vi "Read Callibration Datas.vi"(8 "error in (no error)":errorcluster, 11 "file (use dialog)":path=path "D:/WeiFu/Labview ATS/Corner Radar/EOL Test/Corner EOL Radar ATS/SubVi/C Lib/20250509/data_.txt") -> (0 "error out":errorcluster, 3 "Datas":T1[](array[typedef]))   [LabVIEW 2024]
uses:
  Controls/calculate_doa_struct.ctl
  Controls/ant re&im.ctl
  Controls/Calc Para_int.ctl
  Controls/Calc Para_float.ctl
panel:
  out "Numeric":i32
  out "array type (2D Dbl) 2":dbl[](array[numeric])
  out "array type (2D Dbl)":dbl[][](array[numeric])
  out "size(s)":i32
  out "x/y":dbl
  out "array":dbl[](array[numeric])
  out "text":string
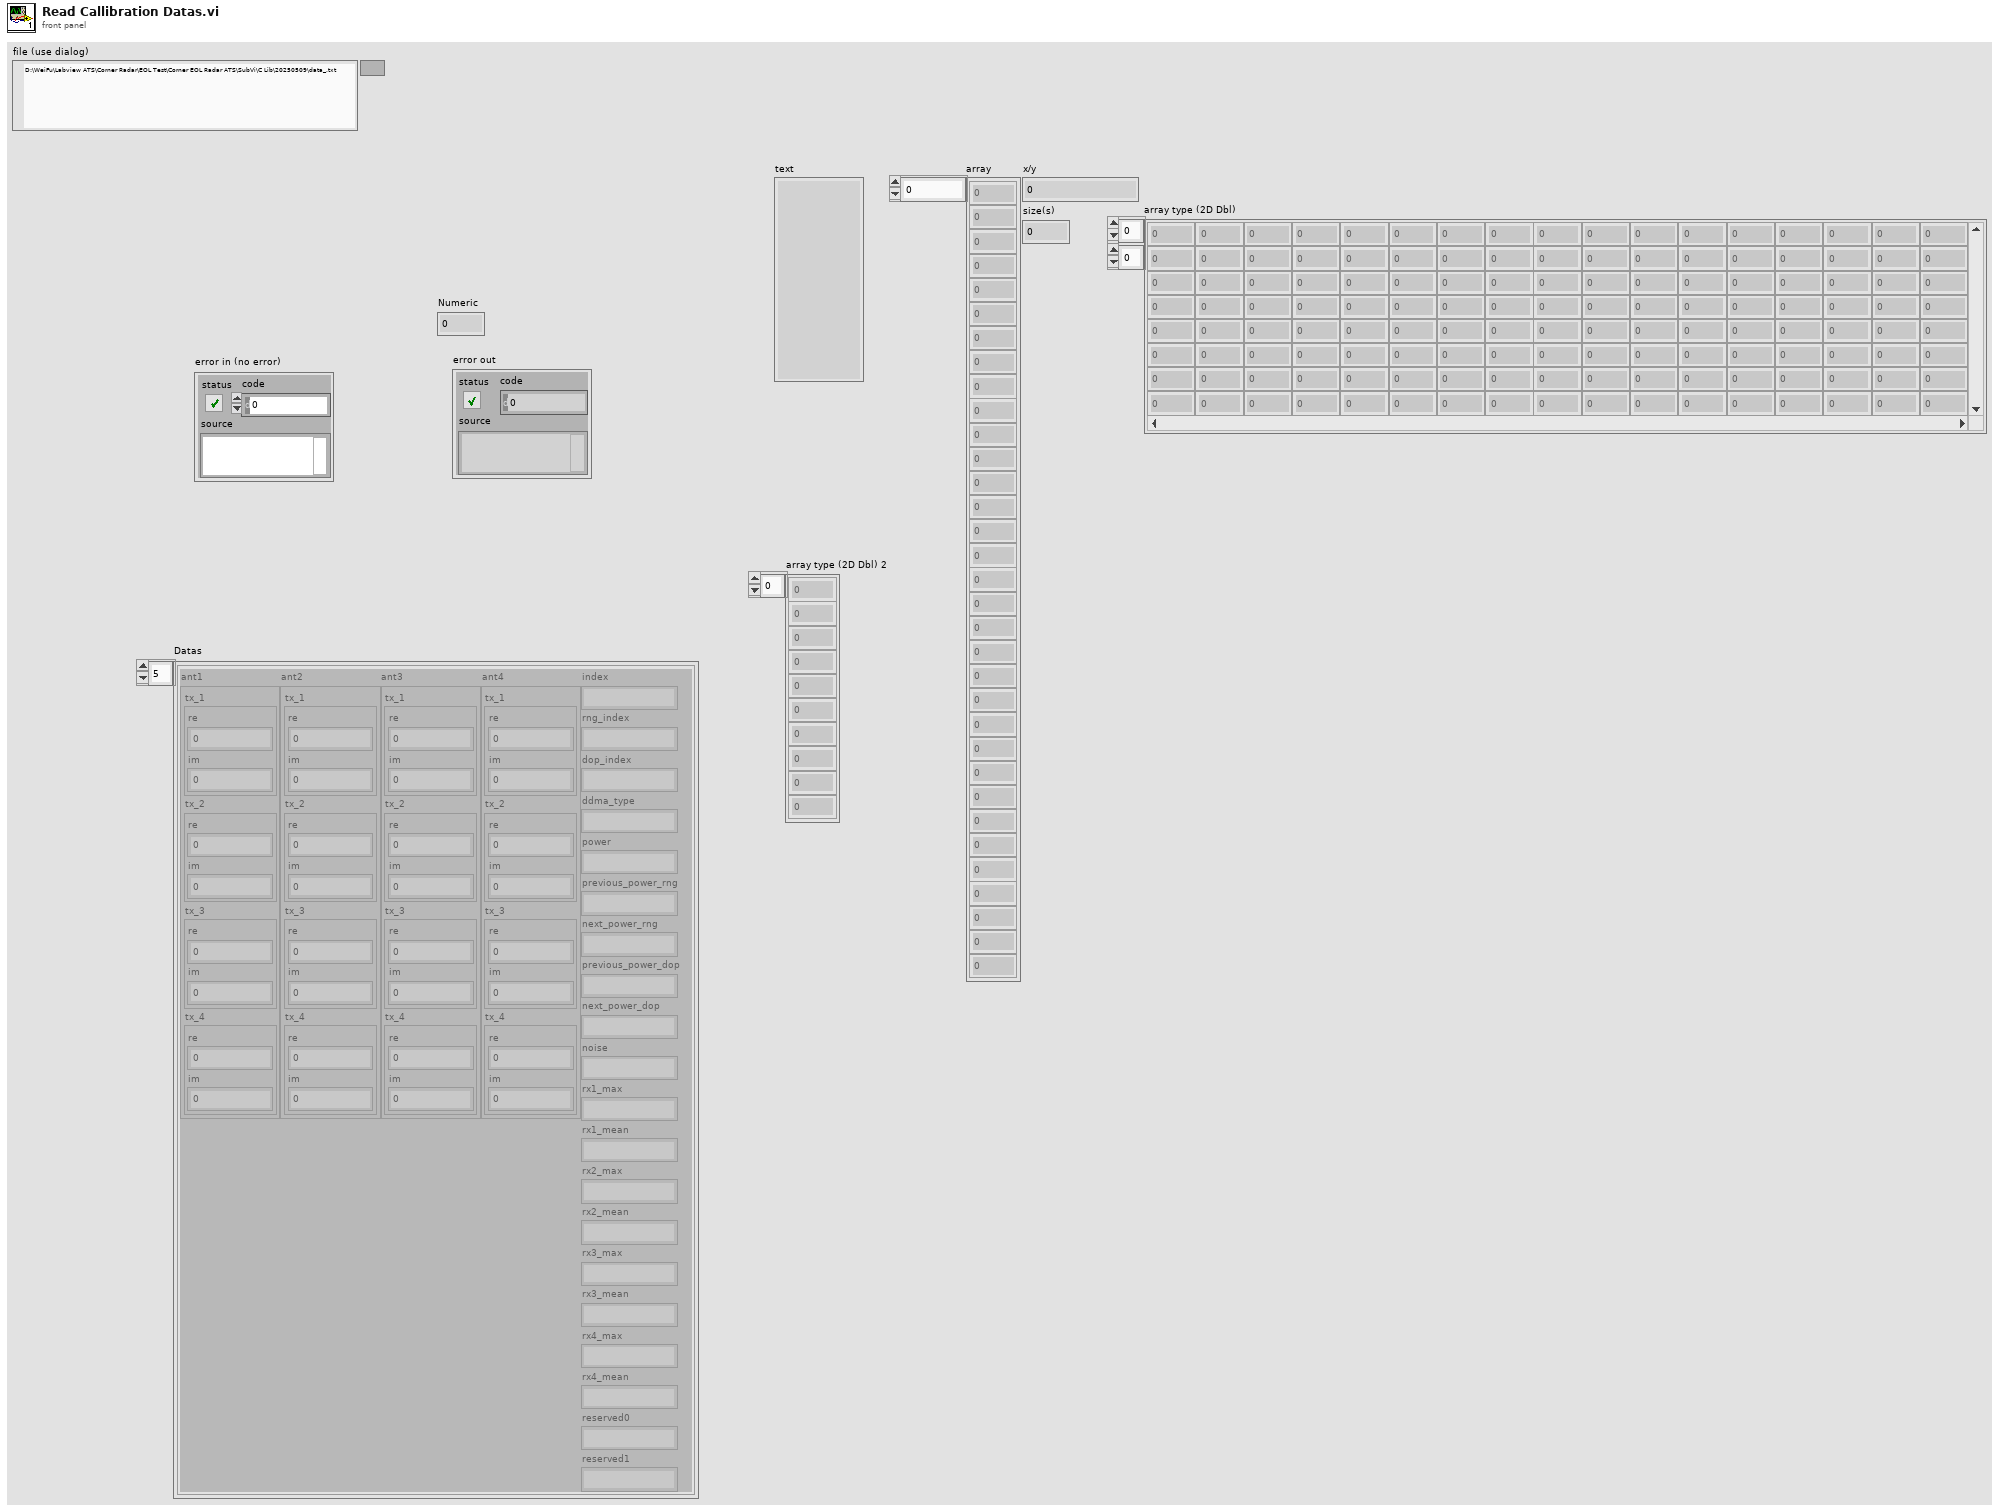
[diagram p1: front panel]
types:
  T1 = typedef "calculate_doa_struct.ctl" = cluster{"ant1":T2, "ant2":T2, "ant3":T2, "ant4":T2, "index":u16, "rng_index":u16, "dop_index":u16, "ddma_type":u16, "power":u32, "previous_power_rng":u32, "next_power_rng":u32, "previous_power_dop":u32, "next_power_dop":u32, "noise":u32, "rx1_max":u32, "rx1_mean":u32, "rx2_max":u32, "rx2_mean":u32, "rx3_max":u32, "rx3_mean":u32, "rx4_max":u32, "rx4_mean":u32, "reserved0":u32, "reserved1":u32}
  T2 = typedef "ant re&im.ctl" = cluster{"tx_1":T3, "tx_2":T3, "tx_3":T3, "tx_4":T3}
  T3 = typedef "Calc Para_int.ctl" = cluster{"re":i32, "im":i32}
  T4 = cluster{"tx_0":T3, "tx_1":T3, "tx_2":T3, "tx_3":T3}
  T5 = typedef "Calc Para_float.ctl" = cluster{"re":sgl, "im":sgl}
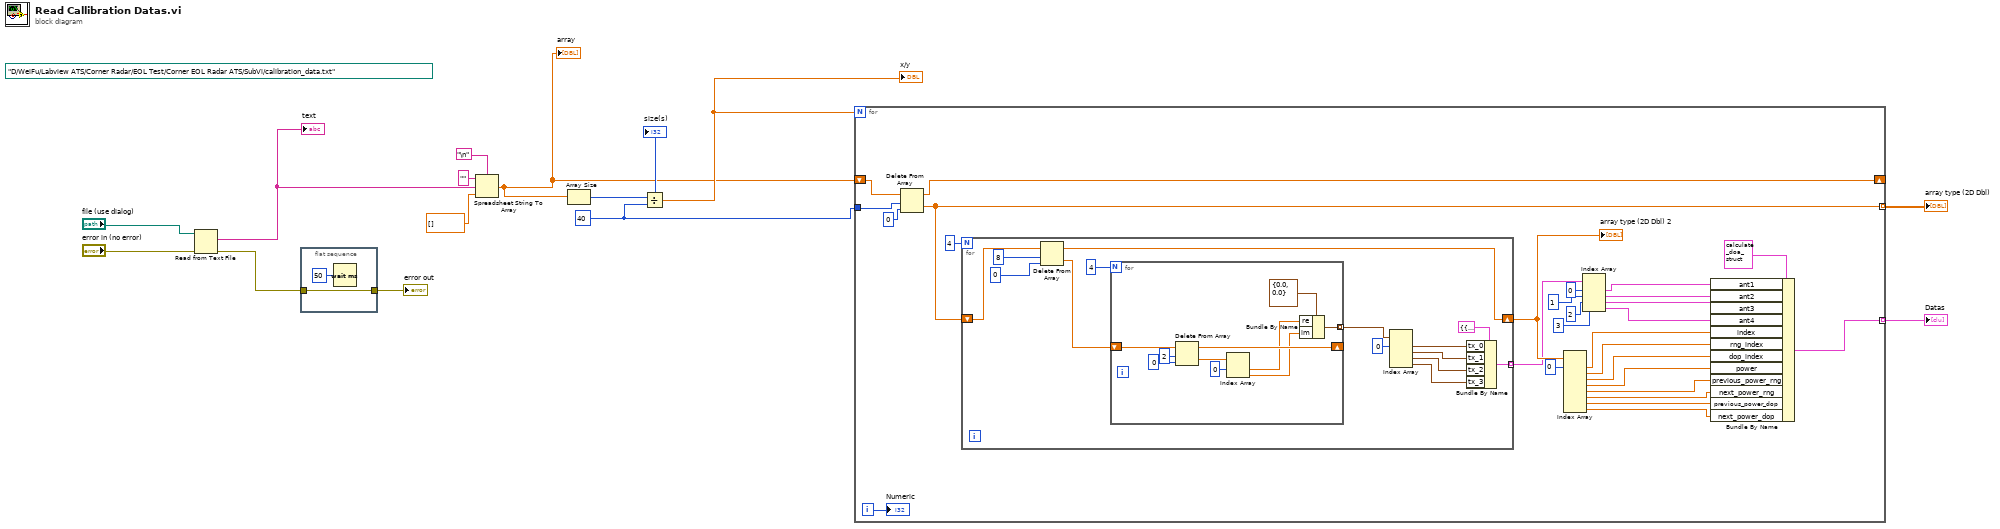
[diagram p0: block diagram]
diagram:
  w7 = 40 ("y")
  (unwired) path "D:/WeiFu/Labview ATS/Corner Radar/EOL Test/Corner EOL Radar ATS/SubVi/calibration_data.txt" ("file (use dialog)")
  n1 = Read from Text File(file (use dialog)="file (use dialog)", error in="error in (no error)") -> (text=w14:string, error out=w3:errorcluster)  [unwired: 2 in, 2 out]
  "text" <- w14
  n2 = flat-sequence {
    tunnel: w3 -> [w15]
    tunnel: [w15] -> w1
    frame #0 {
      n3 = Wait (ms)(milliseconds to wait=u32 50) -> ()  [unwired: 1 out]
    }
  }
  n4 = Spreadsheet String To Array(delimiter (Tab)="\n", format string="", spreadsheet string=w14, array type (2D Dbl)=dbl[] []) -> (array=w8:dbl[])
  "array" <- w8
  n5 = Array Size(array=w8) -> (size(s)=w10:i32)
  "size(s)" <- w10
  n6 = Divide(x=w10, y=w7) -> (x/y=w9:dbl)
  "x/y" <- w9
  n7 = for {
    N: w9 -> [_]
    shift-right: [w41] -> _
    shift-left: w8 -> [w44]
    tunnel: w7 -> [w43]
    tunnel: [w39] -> w6 mode=indexing
    tunnel: [w40] -> w5 mode=indexing
    i -> [w17]
    n8 = Delete From Array(array=w44, length=w43, index=0) -> (deleted portion=w39:dbl[], array with subset deleted=w41:dbl[])
    n9 = for {
      N: 4 -> [_]
      shift-right: [w55] -> w38
      shift-left: w39 -> [w56]
      tunnel: [w46] -> w35 mode=indexing
      n10 = Delete From Array(array=w56, length=8, index=0) -> (deleted portion=w53:dbl[], array with subset deleted=w55:dbl[])
      n11 = for {
        N: 4 -> [_]
        shift-right: [w65] -> _
        shift-left: w53 -> [w68]
        tunnel: [w60] -> w48 mode=indexing
        n12 = Delete From Array(array=w68, length=2, index=0) -> (deleted portion=w64:dbl[], array with subset deleted=w65:dbl[])
        n13 = Index Array(array=w64, index #1=0 ("index")) -> (element #1=w62:dbl, element #2=w61:dbl)  [unwired: 1 in]
        n14 = Bundle By Name(cluster=T5 {"re"=0.0, "im"=0.0} ("calibration_parameters"), "re"=w62, "im"=w61) -> (w60:T5)
      }
      n15 = Index Array(array=w48, index #1=0 ("index")) -> (element #1=w47:T5, element #2=w50:T5, element #3=w51:T5, element #4=w52:T5)  [unwired: 3 in]
      n16 = Bundle By Name(cluster=T4 {"tx_0"={"re"=0, "im"=0}, "tx_1"={"re"=0, "im"=0}, "tx_2"={"re"=0, "im"=0}, "tx_3"={"re"=0, "im"=0}} ("element"), "tx_0"=w47, "tx_1"=w50, "tx_2"=w51, "tx_3"=w52) -> (w46:T4)
    }
    "array type (2D Dbl) 2" <- w38
    n17 = Index Array(array=w38, index #1=0 ("index")) -> (element #1=w30:dbl, element #2=w29:dbl, element #3=w28:dbl, element #4=w22:dbl, element #5=w21:dbl, element #6=w20:dbl, element #7=w19:dbl, element #8=w18:dbl)  [unwired: 7 in]
    n18 = Index Array(array=w35, index #1=0 ("index (row)"), index #2=1 ("index (row)"), index #3=2 ("index (row)"), index #4=3 ("index (row)")) -> (element #1=w27:T4, element #2=w26:T4, element #3=w25:T4, element #4=w24:T4)
    n19 = Bundle By Name(cluster=T1 {"ant1"={"tx_1"={"re"=0, "im"=0}, "tx_2"={"re"=0, "im"=0}, "tx_3"={"re"=0, "im"=0}, "tx_4"={"re"=0, "im"=0}}, "ant2"={"tx_1"={"re"=0, "im"=0}, "tx_2"={"re"=0, "im"=0}, "tx_3"={"re"=0, "im"=0}, "tx_4"={"re"=0, "im"=0}}, "ant3"={"tx_1"={"re"=0, "im"=0}, "tx_2"={"re"=0, "im"=0}, "tx_3"={"re"=0, "im"=0}, "tx_4"={"re"=0, "im"=0}}, "ant4"={"tx_1"={"re"=0, "im"=0}, "tx_2"={"re"=0, "im"=0}, "tx_3"={"re"=0, "im"=0}, "tx_4"={"re"=0, "im"=0}}, "index"=2, "rng_index"=20, "dop_index"=215, "ddma_type"=0, "power"=0, "previous_power_rng"=0, "next_power_rng"=0, "previous_power_dop"=0, "next_power_dop"=0, "noise"=0, "rx1_max"=0, "rx1_mean"=0, "rx2_max"=0, "rx2_mean"=0, "rx3_max"=0, "rx3_mean"=0, "rx4_max"=0, "rx4_mean"=0, "reserved0"=0, "reserved1"=0} ("Calculate_doa_data"), "ant1"=w27, "ant2"=w26, "ant3"=w25, "ant4"=w24, "index"=w30, "rng_index"=w29, "dop_index"=w28, "power"=w22, "previous_power_rng"=w21, "next_power_rng"=w20, "previous_power_dop"=w19, "next_power_dop"=w18) -> (w40:T1)
    "Numeric" <- w17
  }
  "array type (2D Dbl)" <- w6
  "Datas" <- w5
  "error out" <- w1
